vi "Create_Heater_Setpoints_File.vi"(4 "Mode":enum16{"Load from File", "Save to File"}(ring), 8 "Filename":path) -> ()   [LabVIEW 2010]
uses:
  ADAM Client/Sub VIs/Heater_Setpoint.ctl
panel:
  out "Setpoints Out":T1[](array[typedef])
  in  "Setpoints In":T1[](array[typedef])
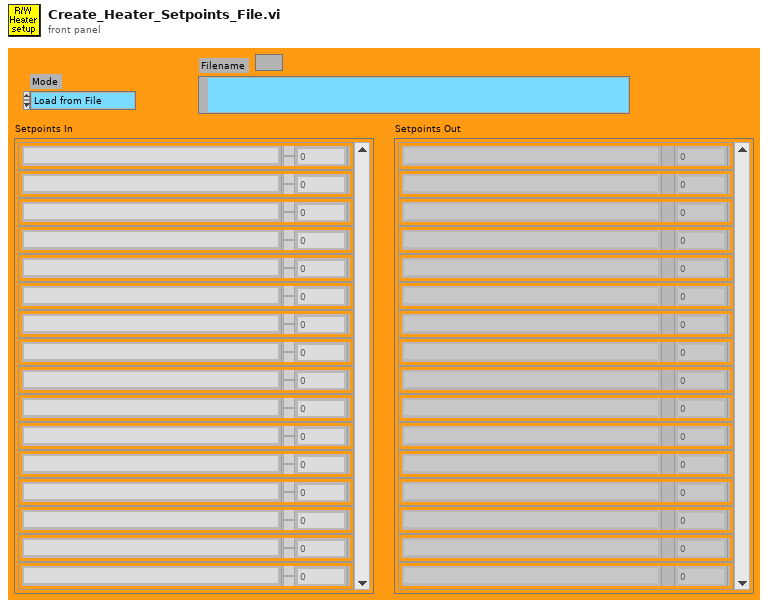
[diagram p1: front panel]
types:
  T1 = typedef "Heater_Setpoint.ctl" = cluster{"Ch Name":string, "Setpoint":dbl}
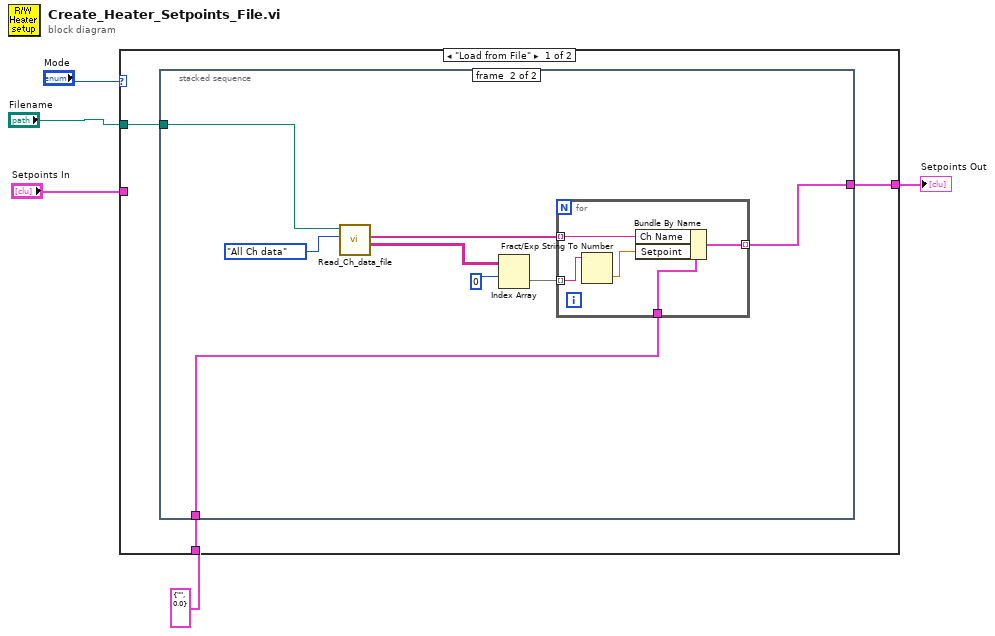
[diagram p0: block diagram]
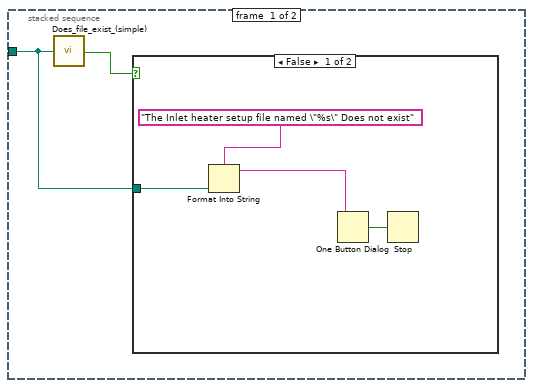
[diagram p2: hidden frame]
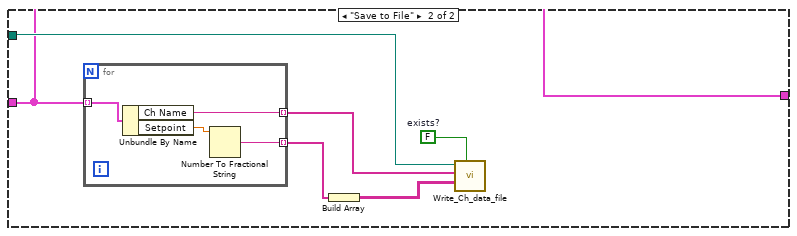
[diagram p4: hidden frame]
diagram:
  n1 = case shown="\"Load from File\"" "Mode" {
    tunnel: "Filename" -> [w8 w33]
    tunnel: T1 {"Ch Name"="", "Setpoint"=0.0} ("Cluster") -> [w7 _]
    tunnel: [w6 w28] -> w2
    tunnel: "Setpoints In" -> [_ w28]
    frame "Load from File" {
      n2 = stacked-sequence {
        tunnel: w8 -> [w9 w17]
        tunnel: w7 -> [_ w21]
        tunnel: [_ w19] -> w6
        frame #0 {
          n3 = call "Does_file_exist_(simple).vi"("Pathname"=w9) -> ("exists?"=w10:bool)
          n4 = case shown="False" w10 {
            tunnel: w9 -> [w14 _]
            frame False {
              n5 = Format Into String(format string="The Inlet heater setup file named \"%s\" Does not exist" ("Format String"), w14) -> (resulting string=w13:string)  [unwired: 2 in, 1 out]
              n6 = One Button Dialog(message=w13) -> (true=w11:bool)  [unwired: 1 out]
              n7 = Stop(stop? (T)=w11) -> ()
            }
            frame True {
            }
          }
        }
        frame #1 {
          n8 = call "Read_Ch_data_file.vi"("Output"=enum16{"All Ch data", "The last few rows"}."All Ch data", "Filename"=w17) -> ("Channel Values"=w15:string[][], "Merged Channels"=w16:string[])  [unwired: 3 in, 3 out]
          n9 = Index Array(array=w15, index (row)=0 ("Index")) -> (element=w20:string[])  [unwired: 1 in]
          n10 = for {
            tunnel: w21 -> [w27]
            tunnel: w16 -> [w26] mode=indexing
            tunnel: w20 -> [w25] mode=indexing
            tunnel: [w23] -> w19 mode=indexing
            n11 = Fract/Exp String To Number(string=w25) -> (number=w24:dbl)  [unwired: 4 out]
            n12 = Bundle By Name(cluster=w27, "Ch Name"=w26, "Setpoint"=w24) -> (w23:T1)
          }
        }
      }
    }
    frame "Save to File" {
      w32 = FALSE  # exists?
      n13 = for {
        tunnel: w28 -> [w37] mode=indexing
        tunnel: [w35] -> w30 mode=indexing
        tunnel: [w34] -> w29 mode=indexing
        n14 = Unbundle By Name(w37) -> ("Ch Name"=w34:string, "Setpoint"=w36:dbl)
        n15 = Number To Fractional String(number=w36) -> (F-format string=w35:string)  [unwired: 3 out]
      }
      n16 = Build Array(w30) -> (w31:string[][])
      n17 = call "Write_Ch_data_file.vi"("exists?"=w32, "Channel Values"=w31, "Channel names"=w29, "Filename"=w33) -> ()  [unwired: 4 in, 4 out]
    }
  }
  "Setpoints Out" <- w2
